vi "Configure Fault Location Gating Distance.vi"(0 "VISA resource name":refnum<visa-resource-name>, 1 "Channel (1)":i32=1, 2 "Gating Function State (F: Disable)":bool, 3 "Unit (0: Meter)":u16(ring) items=["Meter", "Feet"], 5 "Gate Type (0: Band-pass)":u16(ring) items=["Band-pass", "Notch"], 7 "Gate Shape (2: Normal Shape)":u16(ring)=2 items=["Maximum Shape", "Wide Shape", "Normal Shape", "Minimum Shape"], 9 "Setting Type (1: Start/Stop)":u16(ring)=1 items=["Center/Span", "Start/Stop"], 11 "error in (no error)":errorcluster, 12 "Start / Center (0.0)":dbl format="%^.2e", 13 "Stop / Span (1.0E-8)":dbl=1e-08 format="%.2g") -> (4 "VISA resource name out":refnum<visa-resource-name>, 15 "error out":errorcluster)   [LabVIEW 2022 SP3, in "Agilent ENA Series.lvlib"]
doc: "Configures the time domain gating distance.\n\n<B>Note:</B> \nThis VI is only valid on E5061B"
uses:
  <instrlib>/Agilent ENA Series/Agilent ENA Series.lvlib
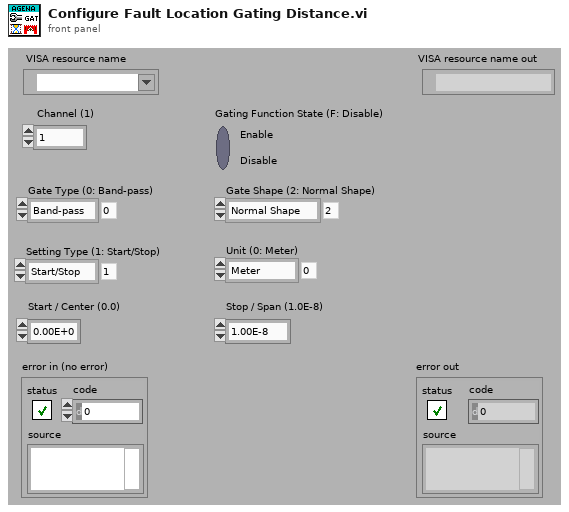
[diagram p1: front panel]
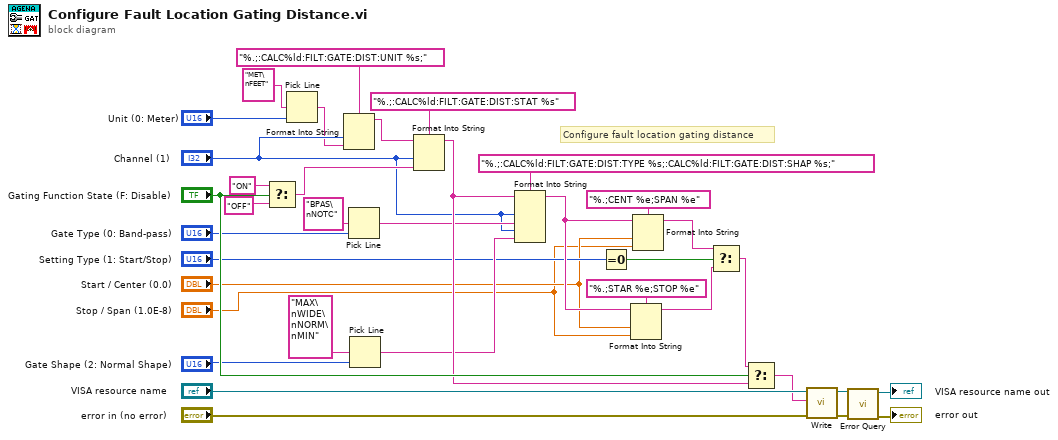
[diagram p0: block diagram]
diagram:
  # "Configure fault location gating distance"
  n1 = Select(t="ON", s="Gating Function State (F: Disable)", f="OFF") -> (s? t:f=w31:string)
  n2 = Pick Line(multi-line string="MET\nFEET", line index="Unit (0: Meter)") -> (output string=w3:string)  [unwired: 1 in]
  n3 = Format Into String(format string="%.;:CALC%ld:FILT:GATE:DIST:UNIT %s;", "Channel (1)", w3) -> (resulting string=w1:string)  [unwired: 2 in, 1 out]
  n4 = Pick Line(multi-line string="BPAS\nNOTC", line index="Gate Type (0: Band-pass)") -> (output string=w25:string)  [unwired: 1 in]
  n5 = Pick Line(multi-line string="MAX\nWIDE\nNORM\nMIN", line index="Gate Shape (2: Normal Shape)") -> (output string=w24:string)  [unwired: 1 in]
  n6 = Format Into String(format string="%.;:CALC%ld:FILT:GATE:DIST:STAT %s", initial string=w1, "Channel (1)", w31) -> (resulting string=w28:string)  [unwired: 1 in, 1 out]
  n7 = Format Into String(format string="%.;:CALC%ld:FILT:GATE:DIST:TYPE %s;:CALC%ld:FILT:GATE:DIST:SHAP %s;", initial string=w28, "Channel (1)", w25, "Channel (1)", w24) -> (resulting string=w21:string)  [unwired: 1 in, 1 out]
  n8 = Equal To 0?(x="Setting Type (1: Start/Stop)") -> (x = 0?=w20:bool)
  n9 = Format Into String(format string="%.;STAR %e;STOP %e", initial string=w21, "Start / Center (0.0)", "Stop / Span (1.0E-8)") -> (resulting string=w18:string)  [unwired: 1 in, 1 out]
  n10 = Format Into String(format string="%.;CENT %e;SPAN %e", initial string=w21, "Start / Center (0.0)", "Stop / Span (1.0E-8)") -> (resulting string=w19:string)  [unwired: 1 in, 1 out]
  n11 = Select(t=w19, s=w20, f=w18) -> (s? t:f=w17:string)
  n12 = Select(t=w17, s="Gating Function State (F: Disable)", f=w28) -> (s? t:f=w16:string)
  n13 = call <instrlib>:"Write.vi"("error in (no error)"="error in (no error)", "String ()"=w16, "VISA resource name"="VISA resource name") -> ("error out"=w9:errorcluster, "VISA resource name out"=w10:refnum<visa-resource-name>)  [unwired: 6 in, 1 out]
  n14 = call <instrlib>:"Error Query.vi"("error in (no error)"=w9, "VISA resource name"=w10) -> ("error out"=→"error out":errorcluster, "VISA resource name out"=→"VISA resource name out":refnum<visa-resource-name>)  [unwired: 6 in, 2 out]
